vi "Set up VICI.vi"() -> ()   [LabVIEW 2018, in "VICI M6 M50 Party Mode.lvlib"]
uses:
  <vilib>/Instr/_visa.llb/VISA Configure Serial Port (Instr).vi
  VICI M6 M50 Party Mode.lvlib
panel:
  in  "stop":bool
  out "read buffer 4":string
  out "Bytes at Port 5":u32
  out "read buffer 3":string
  out "Bytes at Port 4":u32
  out "String 2":string
  in  "Enum":enum16{"Enter", "Ctrl+J"}(ring)=enum."Ctrl+J"
  in  "message":string
  out "error out":errorcluster
  out "VISA resource name out":refnum<visa-resource-name>
  in  "VISA resource name":refnum<visa-resource-name>
  in  "error in (no error)":errorcluster
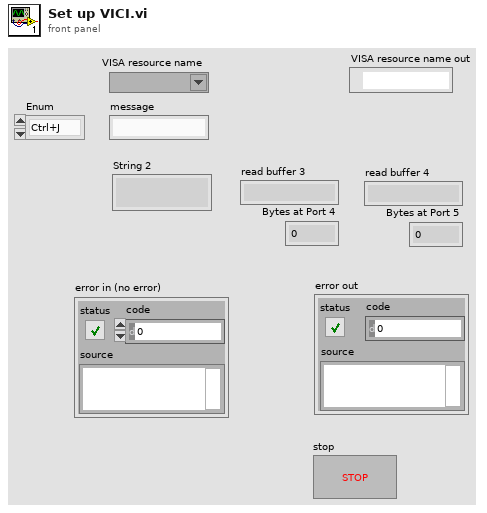
[diagram p1: front panel]
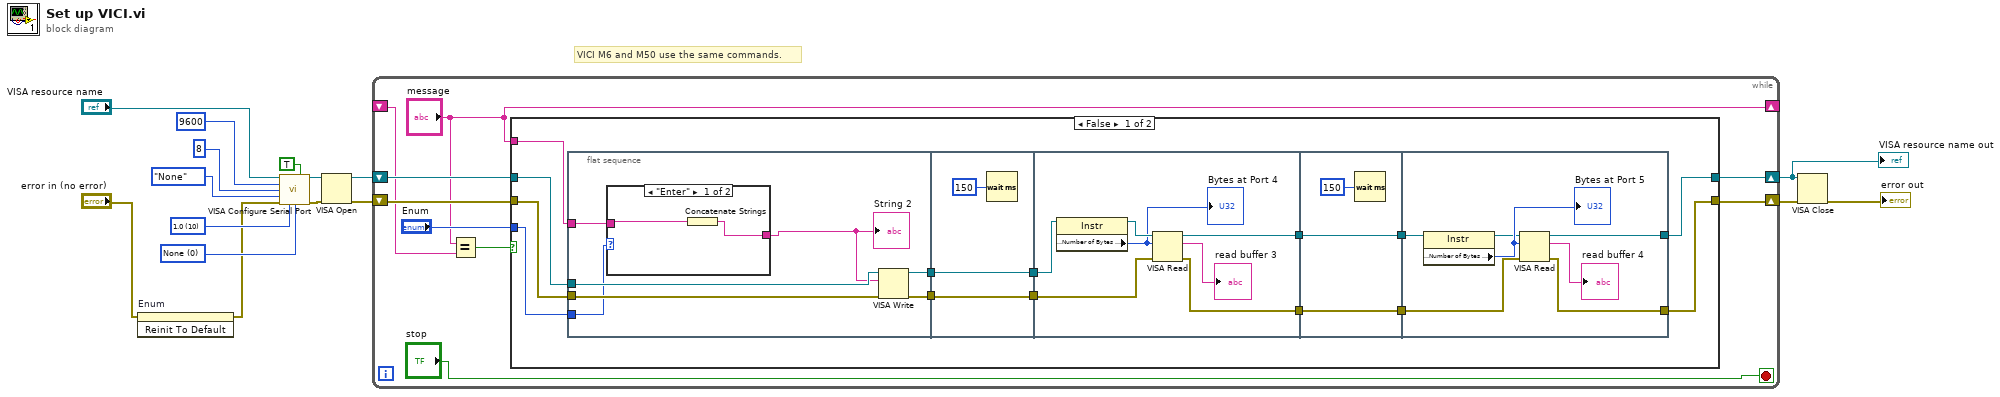
[diagram p0: block diagram]
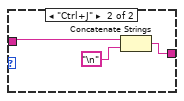
[diagram p2: hidden frame]
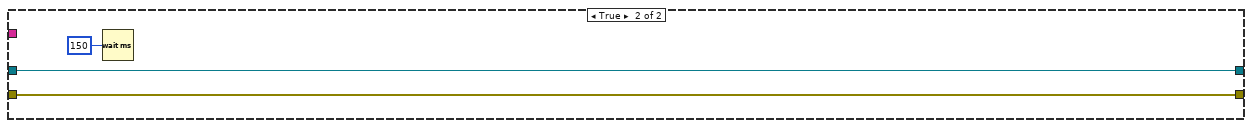
[diagram p3: hidden frame]
diagram:
  w9 = u16 0 items=["None", "XON/XOFF", "RTS/CTS", "XON/XOFF & RTS/CTS", "DTR/DSR", "XON/XOFF & DTR/DSR"] ("flow control (0:none)")
  w10 = u16 10 items=["1.0"=10, "1.5"=15, "2.0"=20] ("stop bits (10: 1 bit)")
  # "VICI M6 and M50 use the same commands."
  n1 = invoke on="Enum" class="Enum (strict)" method="Reinit To Default"(error in="error in (no error)") -> (error out=w2:errorcluster)  [unwired: 2 in, 2 out]
  n2 = call-poly "VISA Configure Serial Port"("VISA resource name"="VISA resource name", "Enable Termination\nChar (T)"=TRUE ("Enable Termination\nChar (T)"), "baud rate (9600)"=u32 9600, "data bits (8)"=u16 8, "parity (0:none)"=enum16{"None", "Odd", "Even", "Mark", "Space"}."None", "error in (no error)"=w2, "stop bits (10: 1 bit)"=w10, "flow control (0:none)"=w9) -> ("VISA resource name out"=w15:refnum<visa-resource-name>, "error out"=w14:errorcluster)  [unwired: 6 in]
  n3 = VISA Open(error in (no error)=w14, VISA resource name=w15) -> (VISA resource name=w7:refnum<visa-resource-name>, error out=w8:errorcluster)  [unwired: 3 in]
  n4 = while {
    shift-right: [w23] -> w5
    shift-left: w8 -> [w25]
    shift-right: [w22] -> w4
    shift-left: w7 -> [w24]
    shift-right: ["message"] -> _
    shift-left: _ -> [w18]
    stop <- "stop" stop-if-true
    n5 = Equal?(x="message", y=w18) -> (x = y?=w20:bool)
    n6 = case shown="False" w20 {
      tunnel: w25 -> [w31 w72]
      tunnel: w24 -> [w30 w73]
      tunnel: "message" -> [w29 _]
      tunnel: [w28 w72] -> w23
      tunnel: [w27 w73] -> w22
      tunnel: "Enum" -> [w26 _]
      frame False {
        n7 = flat-sequence {
          tunnel: w30 -> [w46]
          tunnel: w29 -> [w45]
          tunnel: w31 -> [w44]
          tunnel: [w43] -> w39
          tunnel: [w42] -> w38
          tunnel: w26 -> [w40]
          tunnel: [w54] -> w37
          tunnel: w39 -> [w54]
          tunnel: [w53] -> w36
          tunnel: w38 -> [w53]
          tunnel: w37 -> [w58]
          tunnel: w36 -> [w57]
          tunnel: [w56] -> w35
          tunnel: [w55] -> w34
          tunnel: w35 -> [w64]
          tunnel: [w64] -> w33
          tunnel: w34 -> [w63]
          tunnel: [w63] -> w32
          tunnel: w33 -> [w68]
          tunnel: w32 -> [w67]
          tunnel: [w66] -> w27
          tunnel: [w65] -> w28
          frame #0 {
            n8 = case shown="\"Enter\"" w40 {
              tunnel: w45 -> [w48 w51]
              tunnel: [w47 w50] -> w41
              frame "Enter" {
                n9 = Concatenate Strings(w48) -> (w47:string)
              }
              frame "Ctrl+J" {
                n10 = Concatenate Strings(w51, "\n") -> (w50:string)
              }
            }
            "String 2" <- w41
            n11 = VISA Write(VISA resource name=w46, write buffer=w41, error in (no error)=w44) -> (VISA resource name out=w43:refnum<visa-resource-name>, error out=w42:errorcluster)  [unwired: 1 out]
          }
          frame #1 {
            n12 = Wait (ms)(milliseconds to wait=u32 150) -> ()  [unwired: 1 out]
          }
          frame #2 {
            n13 = property class="Instr"(reference=w58) -> (reference out=w61:refnum<visa-resource-name>, "Serial Settings:Number of Bytes at Serial Port"=w60:u32)  [unwired: 1 in, 1 out]
            "Bytes at Port 4" <- w60
            n14 = VISA Read(VISA resource name=w61, byte count=w60, error in (no error)=w57) -> (VISA resource name out=w56:refnum<visa-resource-name>, read buffer=→"read buffer 3":string, error out=w55:errorcluster)  [unwired: 1 out]
          }
          frame #3 {
            n15 = Wait (ms)(milliseconds to wait=u32 150) -> ()  [unwired: 1 out]
          }
          frame #4 {
            n16 = property class="Instr"(reference=w68) -> (reference out=w69:refnum<visa-resource-name>, "Serial Settings:Number of Bytes at Serial Port"=w70:u32)  [unwired: 1 in, 1 out]
            "Bytes at Port 5" <- w70
            n17 = VISA Read(VISA resource name=w69, byte count=w70, error in (no error)=w67) -> (VISA resource name out=w66:refnum<visa-resource-name>, read buffer=→"read buffer 4":string, error out=w65:errorcluster)  [unwired: 1 out]
          }
        }
      }
      frame True {
        n18 = Wait (ms)(milliseconds to wait=u32 150) -> ()  [unwired: 1 out]
      }
    }
  }
  "VISA resource name out" <- w4
  n19 = VISA Close(VISA resource name=w4, error in (no error)=w5) -> (error out=→"error out":errorcluster)
